vi "Obtain table from UI.vi"(8 "error in (no error)":errorcluster, 10 "Table":string[][](array[string]), 11 "Turnos in":refnum<class "Turnos.lvclass">) -> (0 "error out":errorcluster, 3 "Turnos out":refnum<class "Turnos.lvclass">)   [LabVIEW 2020, in "Turnos.lvlib" / "Turnos.lvclass"]
uses:
  Turnos.lvclass
  Turnos.lvclass/Turnos.ctl
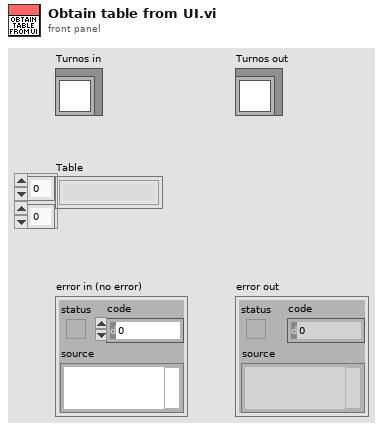
[diagram p1: front panel]
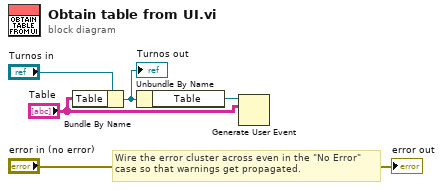
[diagram p0: block diagram]
diagram:
  # "Wire the error cluster across even in the \"No Error\"\ncase so that warnings get propagated."
  n1 = Bundle By Name(cluster="Turnos in", "Table"="Table") -> (w3:refnum<class "Turnos.lvclass">)
  "Turnos out" <- w3
  n2 = Unbundle By Name(w3) -> ("Table"=w2:refnum<user-event>)
  n3 = Generate User Event(user event=w2, event data cluster="Table") -> ()  [unwired: 2 in, 2 out]
  "error out" <- "error in (no error)"
